vi "program_sweep.vi"(8 "error in (no error)":errorcluster, 11 "DL090503StimulatorScaffold in":refnum<class "StimulatorDL090503Scaffold.lvclass">) -> (0 "error out":errorcluster, 3 "DL090503StimulatorScaffold out":refnum<class "StimulatorDL090503Scaffold.lvclass">)   [LabVIEW 2010, in "StimulatorDL090503Scaffold.lvclass"]
uses:
  StimulatorDL090503Scaffold.lvclass
  schedule_entry_cluster.ctl
  common/classes/GenericToplevelComponent/GenericToplevelComponent/common_trigger_enum.ctl
  common/classes/GenericToplevelComponent/GenericToplevelComponent/GenericToplevelComponent.lvclass
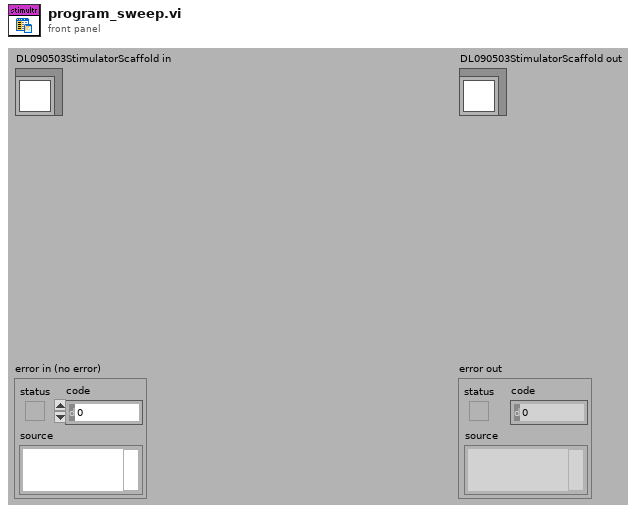
[diagram p1: front panel]
types:
  T1 = typedef "StimulatorDL090503Scaffold.lvclass/schedule_entry_cluster.ctl" = cluster{"time":timestamp, "trigger":T2}
  T2 = typedef "GenericToplevelComponent.lvclass/common_trigger_enum.ctl" = enum16{"NULL", "initialise", "terminate", "fetch command", "fetch data", "attach observer", "register as observer", "detach observer", "acknowledge", "start", "stop", "sweep started", "sweep finished", "experiment started", "experiment stopped"}
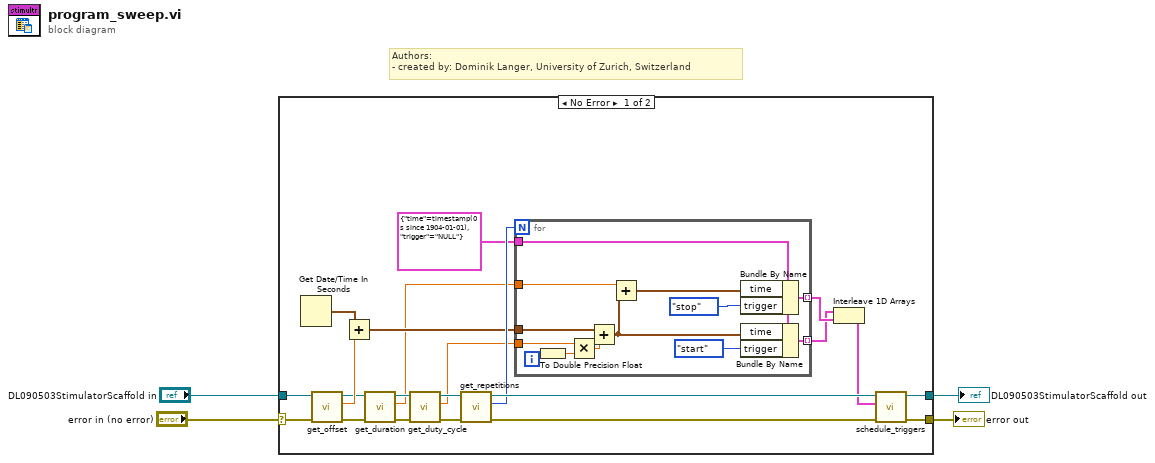
[diagram p0: block diagram]
diagram:
  # "Authors: \n- created by: Dominik Langer, University of Zurich, Switzerland"
  n1 = case shown="No Error" "error in (no error)" {
    selector: "error in (no error)" -> [w24 w41]
    tunnel: [w26 w41] -> w3
    tunnel: [w25 w40] -> w1
    tunnel: "DL090503StimulatorScaffold in" -> [w23 w40]
    frame No Error {
      n2 = Get Date/Time In Seconds() -> (seconds since 1Jan1904=w21:timestamp)
      n3 = call-dynamic "get_offset.vi"("error in (no error)"=w24, "DL090503StimulatorScaffold.lvclass in"=w23) -> ("error out"=w12:errorcluster, "offset"=w22:dbl[unit], "DL090503StimulatorScaffold.lvclass out"=w9:refnum<class "StimulatorDL090503Scaffold.lvclass">)  [unwired: 7 out]
      n4 = Add(x=w21, y=w22) -> (x+y=w13:timestamp)
      n5 = call-dynamic "get_duration.vi"("error in (no error)"=w12, "DL090503StimulatorScaffold.lvclass in"=w9) -> ("error out"=w11:errorcluster, "duration"=w8:dbl[unit], "DL090503StimulatorScaffold.lvclass out"=w10:refnum<class "StimulatorDL090503Scaffold.lvclass">)  [unwired: 7 out]
      n6 = call-dynamic "get_duty_cycle.vi"("error in (no error)"=w11, "DL090503StimulatorScaffold.lvclass in"=w10) -> ("error out"=w16:errorcluster, "duty cycle"=w14:dbl[unit], "DL090503StimulatorScaffold.lvclass out"=w15:refnum<class "StimulatorDL090503Scaffold.lvclass">)  [unwired: 7 out]
      n7 = call-dynamic "get_repetitions.vi"("error in (no error)"=w16, "DL090503StimulatorScaffold.lvclass in"=w15) -> ("error out"=w20:errorcluster, "repetitions"=w18:i32, "DL090503StimulatorScaffold.lvclass out"=w19:refnum<class "StimulatorDL090503Scaffold.lvclass">)  [unwired: 7 out]
      n8 = for {
        N: w18 -> [_]
        tunnel: T1 {"time"=timestamp(0 s since 1904-01-01), "trigger"=enum."NULL"} ("schedule entry") -> [w32]
        tunnel: w14 -> [w39]
        tunnel: w13 -> [w35]
        tunnel: w8 -> [w34]
        tunnel: [w30] -> w6 mode=indexing
        tunnel: [w29] -> w5 mode=indexing
        i -> [w37]
        n9 = To Double Precision Float(number=w37) -> (double precision float=w38:dbl)
        n10 = Multiply(x=w39, y=w38) -> (x*y=w36:dbl[unit])
        n11 = Add(x=w35, y=w36) -> (x+y=w33:timestamp)
        n12 = Add(x=w34, y=w33) -> (x+y=w31:timestamp)
        n13 = Bundle By Name(cluster=w32, "time"=w31, "trigger"=common_trigger_enum."stop") -> (w30:T1)
        n14 = Bundle By Name(cluster=w32, "time"=w33, "trigger"=common_trigger_enum."start") -> (w29:T1)
      }
      n15 = Interleave 1D Arrays(w5, w6) -> (w7:T1[])
      n16 = call-dynamic "schedule_triggers.vi"("error in (no error)"=w20, "new schedule entries"=w7, "DL090503StimulatorScaffold in"=w19) -> ("error out"=w26:errorcluster, "DL090503StimulatorScaffold out"=w25:refnum<class "StimulatorDL090503Scaffold.lvclass">)  [unwired: 7 out]
    }
    frame Error {
    }
  }
  "error out" <- w3
  "DL090503StimulatorScaffold out" <- w1
